vi "Close Session.vi"(0 "eye scan in":refnum<class "niHighSpeedSerial Eye Scan v1 Host.lvclass">, 11 "error in":errorcluster) -> (15 "error out":errorcluster)   [LabVIEW 2014, in "niHighSpeedSerial Eye Scan v1 Host.lvclass"]
doc: "Closes the specified session and frees reserved resources. If the session is running, it is first aborted.\n\n<B>Input Parameters</B>\n\n<B>eye scan in</B> Takes in a reference to your session from the previous VI.\n\n<B>error in</B> describes error conditions that occur before this node runs. This input provides standard 'error in' functionality.\n\n<B>Output Parameters</B>\n\n<B>error out</B> contains error information. This output provides standard 'error out' functionality."
uses:
  <instrlib>/niHighSpeedSerial/Eye Scan/v1/Host/Eye Scan/niHighSpeedSerial Eye Scan v1 Host.lvclass
  <instrlib>/niHighSpeedSerial/Eye Scan/v1/Host/Eye Scan/niHighSpeedSerial Eye Scan v1 Host.lvclass/niHighSpeedSerial Eye Scan v1 Host.ctl
  <instrlib>/_niInstr/Instruction Framework/v1/Host/Instruction Target/niInstr Instruction Target v1 Host.lvclass
  <instrlib>/niHighSpeedSerial/Eye Scan/v1/Host/Impl/Eye Scan Point Iterator/niHighSpeedSerial Eye Scan Point Iterator v1 Host.lvclass
  <instrlib>/niHighSpeedSerial/Eye Scan/v1/Host/Impl/Single Point/niHighSpeedSerial Eye Scan Single Point v1 Host.lvclass
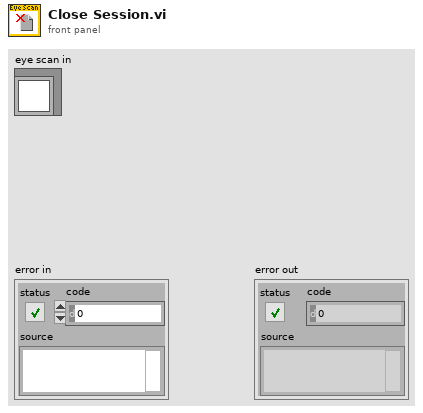
[diagram p1: front panel]
types:
  T1 = typedef "niHighSpeedSerial Eye Scan v1 Host.lvclass/Private Data.ctl" = cluster{"instruction target":refnum<class "niInstr Instruction Target v1 Host.lvclass">, "channels":T2[], "measure state":T3, "rx output divider":T4, "equalization mode":T5, "rx data width":T6, "BER floor":dbl, "number of points completed":i32, "rx output divider configured?":bool, "equalization mode configured?":bool, "rx data width configured?":bool}
  T2 = typedef "niHighSpeedSerial Eye Scan v1 Host.lvclass/Channel Data.ctl" = cluster{"instance":u8, "channel":refnum<class "niHighSpeedSerial Eye Scan Single Point v1 Host.lvclass">, "point iterator":refnum<class "niHighSpeedSerial Eye Scan Point Iterator v1 Host.lvclass">}
  T3 = typedef "niHighSpeedSerial Eye Scan v1 Host.lvclass/Measure State.ctl" = enum16{"Uninitialized", "Initialized", "Ready", "Measuring", "Finished", "Aborted"}
  T4 = typedef "niHighSpeedSerial Eye Scan Common v1 Host.lvlib/RX Output Divider.ctl" = enum16{"1", "2", "4", "8", "16"}
  T5 = typedef "niHighSpeedSerial Eye Scan Common v1 Host.lvlib/Equalization Mode.ctl" = enum16{"DFE", "LPM"}
  T6 = typedef "niHighSpeedSerial Eye Scan Common v1 Host.lvlib/Data Width.ctl" = enum16{"16 Bit", "20 Bit", "32 Bit", "40 Bit"}
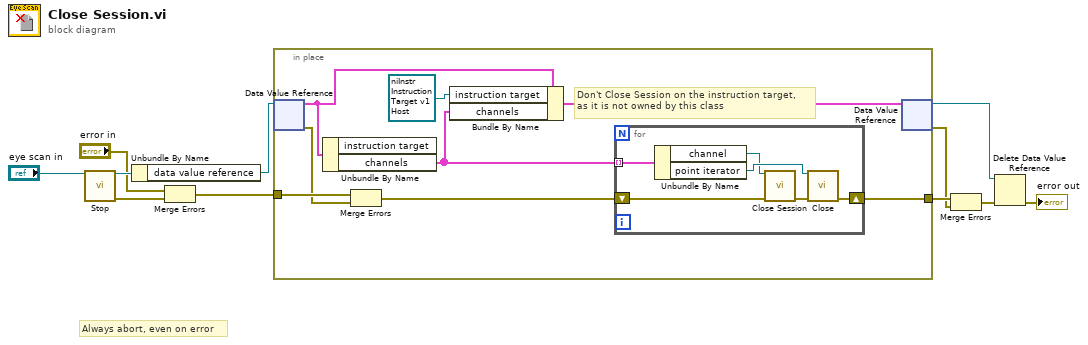
[diagram p0: block diagram]
diagram:
  # "Always abort, even on error"
  n1 = call <instrlib>:"Stop.vi"("eye scan in"="eye scan in") -> ("eye scan out"=w4:refnum<class "niHighSpeedSerial Eye Scan v1 Host.lvclass">, "error out"=w2:errorcluster)  [unwired: 13 in]
  n2 = Unbundle By Name(w4) -> ("data value reference"=w6:refnum<data-value>)
  n3 = Merge Errors("error in", w2) -> (w1:errorcluster)
  n4 = in-place {
    in-place-border: w1 -> [w19]
    in-place-border: [w17] -> w10
    # "Don't Close Session on the instruction target,\nas it is not owned by this class"
    n5 = in-place-dvr #1(w6) -> (w16:T1, w18:errorcluster)
    n6 = Unbundle By Name(w16) -> ("channels"=w13:T2[])  [unwired: 1 out]
    n7 = Merge Errors(w19, w18) -> (w14:errorcluster)
    n8 = Bundle By Name(cluster=w16, "instruction target"=refnum<class "niInstr Instruction Target v1 Host.lvclass"> refnum, "channels"=w13) -> (w15:T1)
    n9 = for {
      tunnel: w13 -> [w20] mode=indexing
      shift-right: [w21] -> w17
      shift-left: w14 -> [w23]
      n10 = Unbundle By Name(w20) -> ("channel"=w24:refnum<class "niHighSpeedSerial Eye Scan Single Point v1 Host.lvclass">, "point iterator"=w25:refnum<class "niHighSpeedSerial Eye Scan Point Iterator v1 Host.lvclass">)
      n11 = call <instrlib>:"Close Session.vi"("eye scan single point"=w24, "error in"=w23) -> ("error out"=w22:errorcluster)  [unwired: 13 in]
      n12 = call-dynamic "Close.vi"("eye scan point iterator"=w25, "error in"=w22) -> ("error out"=w21:errorcluster)  [unwired: 13 in]
    }
    n13 = in-place-dvr #1(w15) -> (w11:refnum<data-value>, w9:errorcluster)
  }
  n14 = Merge Errors(w10, w9) -> (w8:errorcluster)
  n15 = Delete Data Value Reference(data value reference=w11, error in=w8) -> (error out=→"error out":errorcluster)  [unwired: 1 out]
